vi "OC2 Check chxsum.vi"(10 "report string":string) -> (2 "RX packet ok":bool)   [LabVIEW 2009]
uses:
  <vilib>/Utility/error.llb/DialogType.ctl
panel:
  out "length":i32
  out "calc ck":dbl
  in  "error in":errorcluster
  out "read buffer 3":string
  out "SOH FOUND":bool
  out "read cks":dbl
  out "read buffer 2":string
  out "error out":errorcluster
  out "output string":string
  # "Checksum check"
  # "j520.004;0.002;4;4;100.151;100.151;100.000;100.000;1;1;16"
  # "j520.004;0.002;4;4;000.000;100.151;000.000;100.000;0;0;0B"
  # "V1.02"
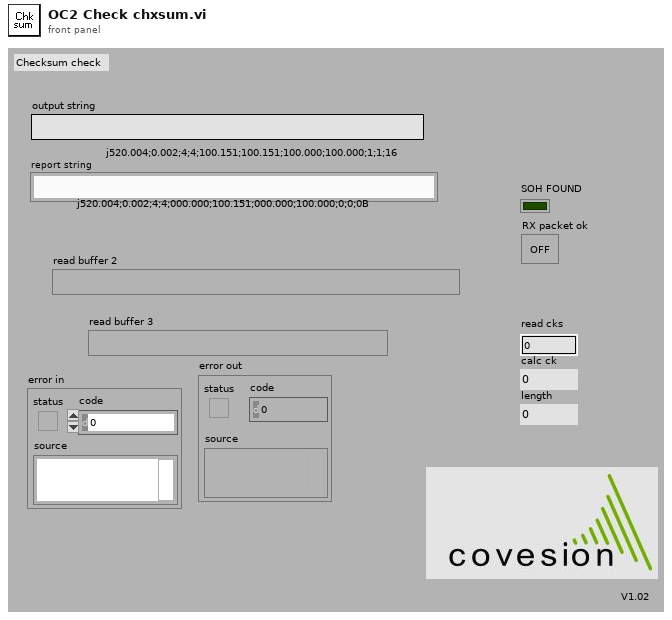
[diagram p1: front panel]
types:
  T1 = typedef "DialogType.ctl" = u16
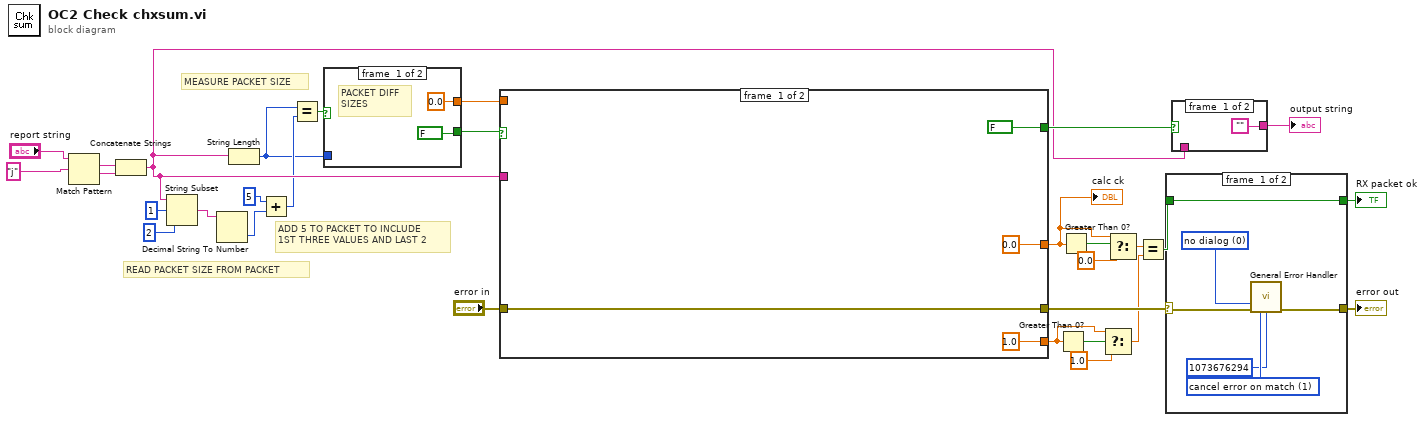
[diagram p0: block diagram]
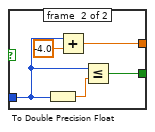
[diagram p2: hidden frame]
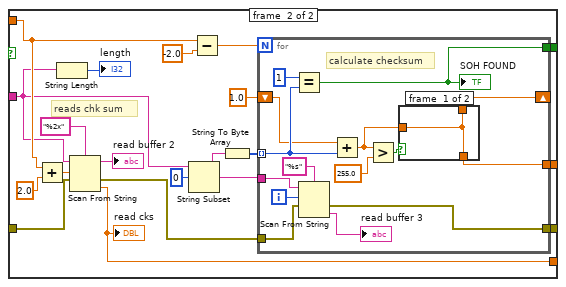
[diagram p4: hidden frame]
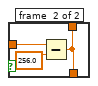
[diagram p5: hidden frame]
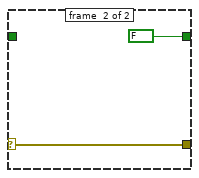
[diagram p6: hidden frame]
diagram:
  # "ADD 5 TO PACKET TO INCLUDE \n1ST THREE VALUES AND LAST 2"
  # "MEASURE PACKET SIZE"
  # "READ PACKET SIZE FROM PACKET"
  n1 = Match Pattern(string="report string", regular expression="j") -> (match substring=w28:string, after substring=w27:string)  [unwired: 1 in, 2 out]
  n2 = Concatenate Strings(w28, w27) -> (w9:string)
  n3 = String Subset(string=w9, offset (0)=1, length (rest)=2 ("length (rest)")) -> (substring=w6:string)
  n4 = Decimal String To Number(string=w6) -> (number=w5:i32)  [unwired: 2 in, 1 out]
  n5 = String Length(string=w9) -> (length=w1:i32)
  n6 = Add(x=5, y=w5) -> (x+y=w2:i32)
  n7 = Equal?(x=w1, y=w2) -> (x = y?=w3:bool)
  n8 = case shown="True" w3 {
    tunnel: [0.0 w37] -> w26
    tunnel: [FALSE w35] -> w25
    tunnel: w1 -> [_ w33]
    frame #0 {
      # "PACKET DIFF\nSIZES"
    }
    frame #1 {
      n9 = To Double Precision Float(number=w33) -> (double precision float=w34:dbl)
      n10 = Add(x=w33, y=-4.0) -> (x+y=w37:dbl)
      n11 = Less Or Equal?(x=w33, y=w34) -> (x <= y?=w35:bool)
    }
  }
  n12 = case shown="True" w25 {
    tunnel: w9 -> [_ w45]
    tunnel: w26 -> [_ w53]
    tunnel: "error in" -> [w41 w47]
    tunnel: [w41 w51] -> w30
    tunnel: [0.0 w50] -> w14
    tunnel: [1.0 ("read cks") w49] -> w15
    tunnel: [FALSE w48] -> w24
    frame #0 {
    }
    frame #1 {
      # "reads chk sum"
      n13 = Add(x=w53, y=2.0) -> (x+y=w54:dbl)
      n14 = String Length(string=w45) -> (length=→"length":i32)
      n15 = Scan From String(format string="%2x", input string=w45, initial scan location=w54, error in=w47) -> (remaining string=→"read buffer 2":string, error out=w46:errorcluster, output 1=w49:dbl)  [unwired: 1 in, 1 out]
      "read cks" <- w49
      n16 = String Subset(string=w45, offset (0)=0) -> (substring=w56:string)  [unwired: 1 in]
      n17 = Subtract(x=w53, y=-2.0) -> (x-y=w43:dbl)
      n18 = String To Byte Array(string=w56) -> (unsigned byte array=w58:u8[])
      n19 = for {
        N: w43 -> [_]
        tunnel: w58 -> [w68] mode=indexing
        tunnel: w56 -> [w72]
        tunnel: [w63] -> w51
        tunnel: [w66] -> w50
        tunnel: [w65] -> w48
        tunnel: w46 -> [w64]
        shift-right: [w61] -> _
        shift-left: 1.0 ("value cks") -> [w62]
        i -> [w69]
        # "calculate checksum"
        n20 = Equal?(x=u8 1, y=w68) -> (x = y?=w65:bool)
        "SOH FOUND" <- w65
        n21 = Scan From String(format string="%s", input string=w72, initial scan location=w69, error in=w64) -> (error out=w63:errorcluster, output 1=→"read buffer 3":string)  [unwired: 1 in, 2 out]
        n22 = Add(x=w62, y=w68) -> (x+y=w74:dbl)
        n23 = Greater?(x=w74, y=255.0) -> (0:w73:bool)
        n24 = case shown="True" w73 {
          tunnel: w74 -> [w76 w79]
          tunnel: [w76 w77] -> w66
          tunnel: [w76 w77] -> w61
          frame #0 {
          }
          frame #1 {
            n25 = Subtract(x=w79, y=256.0) -> (x-y=w77:dbl)
          }
        }
      }
    }
  }
  "calc ck" <- w14
  n26 = Greater Than 0?(x=w15) -> (x > 0?=w16:bool)
  n27 = Greater Than 0?(x=w14) -> (x > 0?=w17:bool)
  n28 = Select(t=w15, s=w16, f=1.0) -> (s? t:f=w12:dbl)
  n29 = Select(t=w14, s=w17, f=0.0) -> (s? t:f=w13:dbl)
  n30 = Equal?(x=w13, y=w12) -> (x = y?=w23:bool)
  n31 = case shown="No Error" w30 {
    selector: w30 -> [w85 w86]
    tunnel: [w80 FALSE] -> w22
    tunnel: [w84 w86] -> w20
    tunnel: w23 -> [w80 _]
    frame #0 {
      w82 = T1 0 items=["no dialog", "OK message", "continue or stop message", "OK message + warnings", "continue/stop + warnings"] ("type of dialog (OK msg:1)")
      w83 = 1 items=["no exception", "cancel error on match", "set error on match"] ("[exception action] (none:0)")
      n32 = call <vilib>:"General Error Handler.vi"("type of dialog (OK msg:1)"=w82, "error in (no error)"=w85, "[exception action] (none:0)"=w83, "[exception code]"=1073676294 ("[error code] (0)")) -> ("error out"=w84:errorcluster)  [unwired: 7 in, 4 out]
    }
    frame #1 {
    }
  }
  "error out" <- w20
  "RX packet ok" <- w22
  n33 = case shown="False" w24 {
    tunnel: w9 -> [_ w89]
    tunnel: ["" ("output string") w89] -> w21
    frame #0 {
    }
    frame #1 {
    }
  }
  "output string" <- w21
